vi "絶対湿度.vi"(1 "温度(℃)":dbl, 2 "水蒸気圧(Pa)":dbl) -> (0 "絶対湿度":dbl)   [LabVIEW 2014]
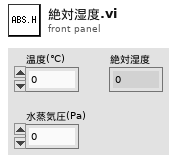
[diagram p1: front panel]
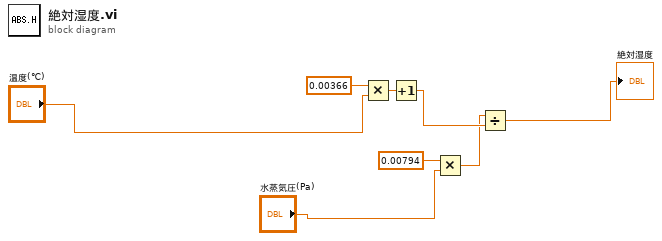
[diagram p0: block diagram]
diagram:
  n1 = Multiply(x=0.00366, y="温度(℃)") -> (x*y=w5:dbl)
  n2 = Increment(x=w5) -> (x+1=w7:dbl)
  n3 = Multiply(x=0.00794, y="水蒸気圧(Pa)") -> (x*y=w6:dbl)
  n4 = Divide(x=w6, y=w7) -> (x/y=→"絶対湿度":dbl)
